vi "Agilent PWM Read Offset Value.vi"(7 "Agilent PWM":T1, 8 "error in (no error)":errorcluster, 11 "VISA Resource Name":refnum<visa-resource-name>) -> (0 "error out":errorcluster, 2 "Value (dB)":dbl, 3 "dup VISA Resource Name":refnum<visa-resource-name>)   [LabVIEW 2011]
doc: "This VI for the HP 8753 is used to read the sweep type.\n\n0 LINEAR FREQ\n1 LOG FREQ\n2 LIST FREQ\n3 CW TIME\n4 POWER SWEEP"
uses:
  TypeDefs/Agilent PWM Instrument Info.ctl
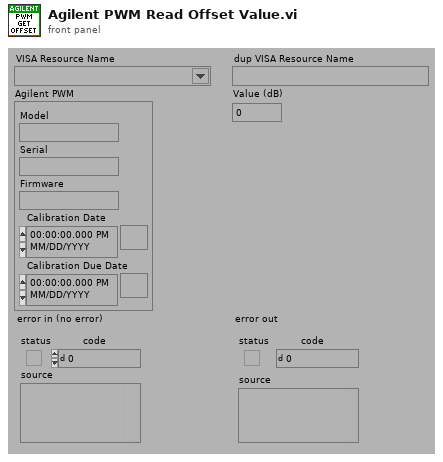
[diagram p1: front panel]
types:
  T1 = typedef "Agilent PWM Instrument Info.ctl" = cluster{"Model":string, "Serial":string, "Firmware":string, "Calibration Date":timestamp, "Calibration Due Date":timestamp}
  T2 = typedef "Agilent PWM Model.ctl" = enum16{"Not Supported", "E4418X", "E4419X", "U2000X"}
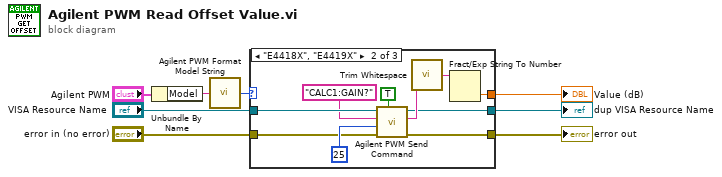
[diagram p0: block diagram]
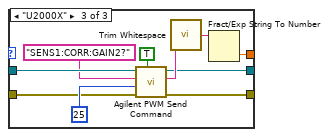
[diagram p3: hidden frame]
diagram:
  n1 = Unbundle By Name("Agilent PWM") -> ("Model"=w7:string)
  n2 = call "Agilent PWM Format Model String.vi"("Model"=w7) -> ("Model"=w6:T2)
  n3 = case shown="\"E4418X\", \"E4419X\"" w6 {
    tunnel: "VISA Resource Name" -> [w10 w17 w27]
    tunnel: [w10 w16 w26] -> w4
    tunnel: [_ w13 w24] -> w3
    tunnel: [w9 w11 w22] -> w1
    tunnel: "error in (no error)" -> [w9 w12 w21]
    frame "Not Supported" {
    }
    frame "E4418X", "E4419X" {
      n4 = call "Agilent PWM Send Command.vi"("Read? (F)"=TRUE, "error in (no error)"=w12, "Byte Count"=u32 25, "Command"="CALC1:GAIN?" ("write buffer"), "VISA Resource Name"=w17) -> ("error out"=w11:errorcluster, "Data Read"=w20:string, "dup VISA Resource Name"=w16:refnum<visa-resource-name>)  [unwired: 4 out]
      n5 = call <vilib>:"Trim Whitespace.vi"("string"=w20) -> ("trimmed string"=w14:string)  [unwired: 1 in]
      n6 = Fract/Exp String To Number(string=w14) -> (number=w13:dbl)  [unwired: 3 in, 1 out]
    }
    frame "U2000X" {
      n7 = call "Agilent PWM Send Command.vi"("Read? (F)"=TRUE, "error in (no error)"=w21, "Byte Count"=u32 25, "Command"="SENS1:CORR:GAIN2?" ("write buffer"), "VISA Resource Name"=w27) -> ("error out"=w22:errorcluster, "Data Read"=w30:string, "dup VISA Resource Name"=w26:refnum<visa-resource-name>)  [unwired: 4 out]
      n8 = call <vilib>:"Trim Whitespace.vi"("string"=w30) -> ("trimmed string"=w23:string)  [unwired: 1 in]
      n9 = Fract/Exp String To Number(string=w23) -> (number=w24:dbl)  [unwired: 3 in, 1 out]
    }
  }
  "dup VISA Resource Name" <- w4
  "error out" <- w1
  "Value (dB)" <- w3
